vi "GOOPUtil_GetParentClassesHiererchy.vi"(8 "error in (no error)":errorcluster, 11 "LabVIEW Object in":refnum<class>) -> (0 "error out":errorcluster, 2 "MyParent  to Parent's Parent order":string[](array[string]), 3 "Array":refnum<class>[](array[class]))   [LabVIEW 2014, in "GOOPUtility.lvlib"]
uses:
  <vilib>/addons/GOOPUtility/GOOPUtility.lvlib
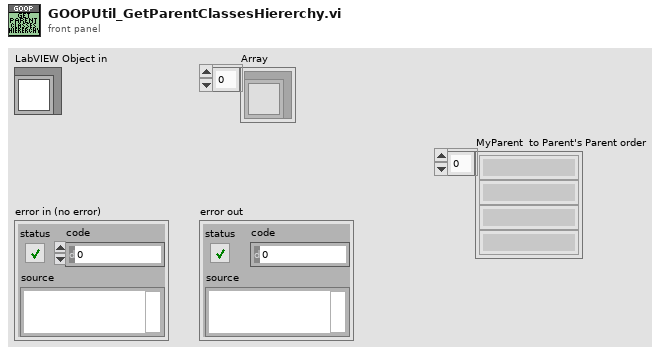
[diagram p1: front panel]
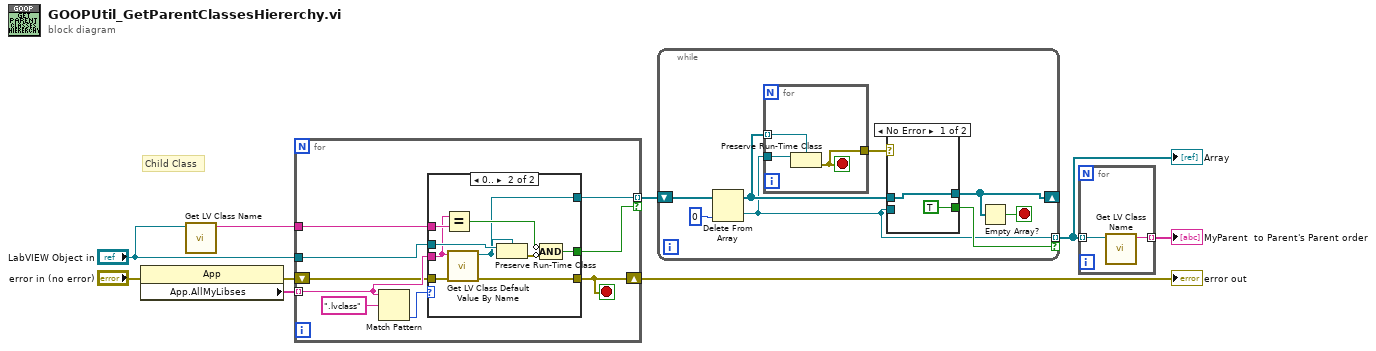
[diagram p0: block diagram]
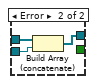
[diagram p2: hidden frame]
diagram:
  # "Child Class"
  n1 = property class="App"(error in="error in (no error)") -> (error out=w3:errorcluster, "App.AllMyLibses"=w2:string[])  [unwired: 1 in, 1 out]
  n2 = call <vilib>:"Get LV Class Name.vi"("object"="LabVIEW Object in") -> ("class name"=w7:string)  [unwired: 9 in, 1 out]
  n3 = for {
    tunnel: w2 -> [w18] mode=indexing
    tunnel: [w13] -> w9 mode=indexing if=w12
    shift-right: [w14] -> w5
    shift-left: w3 -> [w15]
    tunnel: "LabVIEW Object in" -> [w11]
    tunnel: w7 -> [w10]
    stop <- w14 stop-if-true
    n4 = Match Pattern(string=w18, regular expression=".lvclass") -> (offset past match=w17:i32)  [unwired: 1 in, 3 out]
    n5 = case shown="0.." w17 {
      tunnel: [_ w19] -> w13
      tunnel: w18 -> [_ w22]
      tunnel: [_ w27] -> w12
      tunnel: [_ w26] -> w14
      tunnel: w15 -> [_ w25]
      tunnel: w11 -> [_ w24]
      tunnel: w10 -> [_ w23]
      frame Default {
      }
      frame 0.. {
        n6 = Equal?(x=w22, y=w23) -> (x = y?=w21:bool)
        n7 = call <vilib>:"Get LV Class Default Value By Name.vi"("error in (no error)"=w25, "class name"=w22) -> ("error out"=w26:errorcluster, "object"=w19:refnum<class>)  [unwired: 8 in]
        n8 = Preserve Run-Time Class(object in=w24, 2:w19) -> (error out=w20:errorcluster)  [unwired: 1 in, 1 out]
        n9 = Compound Arithmetic op=AND(invert w21, invert w20) -> (w27:bool)
      }
    }
  }
  "error out" <- w5
  n10 = while {
    shift-right: [w28] -> _
    shift-left: w9 -> [w35]
    tunnel: [w29] -> w1 mode=indexing if=w30
    stop <- w32 stop-if-true
    n11 = Delete From Array(array=w35, index=0) -> (deleted portion=w29:refnum<class>, array with subset deleted=w31:refnum<class>[])  [unwired: 1 in]
    n12 = for {
      tunnel: w29 -> [w43]
      tunnel: w31 -> [w42] mode=indexing
      tunnel: [w41] -> w33
      stop <- w41 stop-if-true
      n13 = Preserve Run-Time Class(object in=w43, 2:w42) -> (error out=w41:errorcluster)  [unwired: 1 in, 1 out]
    }
    n14 = case shown="No Error" w33 {
      tunnel: w31 -> [w37 w40]
      tunnel: [w37 w39] -> w28
      tunnel: [TRUE _] -> w30
      tunnel: w29 -> [_ w38]
      frame No Error {
      }
      frame Error {
        n15 = Build Array (concatenate)(w40, w38) -> (w39:refnum<class>[])
      }
    }
    n16 = Empty Array?(array=w28) -> (empty?=w32:bool)
  }
  "Array" <- w1
  n17 = for {
    tunnel: w1 -> [w45] mode=indexing
    tunnel: [w44] -> w8 mode=indexing
    n18 = call <vilib>:"Get LV Class Name.vi"("object"=w45) -> ("class name"=w44:string)  [unwired: 9 in, 1 out]
  }
  "MyParent  to Parent's Parent order" <- w8
